vi "Process.vi"(8 "error in (no error)":errorcluster, 11 "SMO.UI.Example":refnum<class "SMO.UI.Example.lvclass">) -> (0 "error out":errorcluster, 3 "SMO.UI.Example out":refnum<class "SMO.UI.Example.lvclass">)   [LabVIEW 2013, in "SMO.UI.Example.lvclass"]
uses:
  SMO.UI.Example.lvclass
  SMO/Typedefs/Parent Call--Enum.ctl
  SMO.UI.Example.lvclass/SMO.UI.Example.ctl
  SMO.UI/SMO.UI.lvclass
  <vilib>/Utility/miscctls.llb/LVPointTypeDef.ctl
  SMO.Example/SMO.Example.lvclass
  SMO/SMO.lvclass
panel:
  in  "------------ User Events -------":bool=TRUE
  out "Waveform Chart":cluster{"Flow 2":dbl, "Flow 1":dbl}(graph)
  out "Sensor 1 (LPM)":u8
  out "Sensor 2 (LPM)":u8
  in  "Valve":bool
  in  "Pump":bool
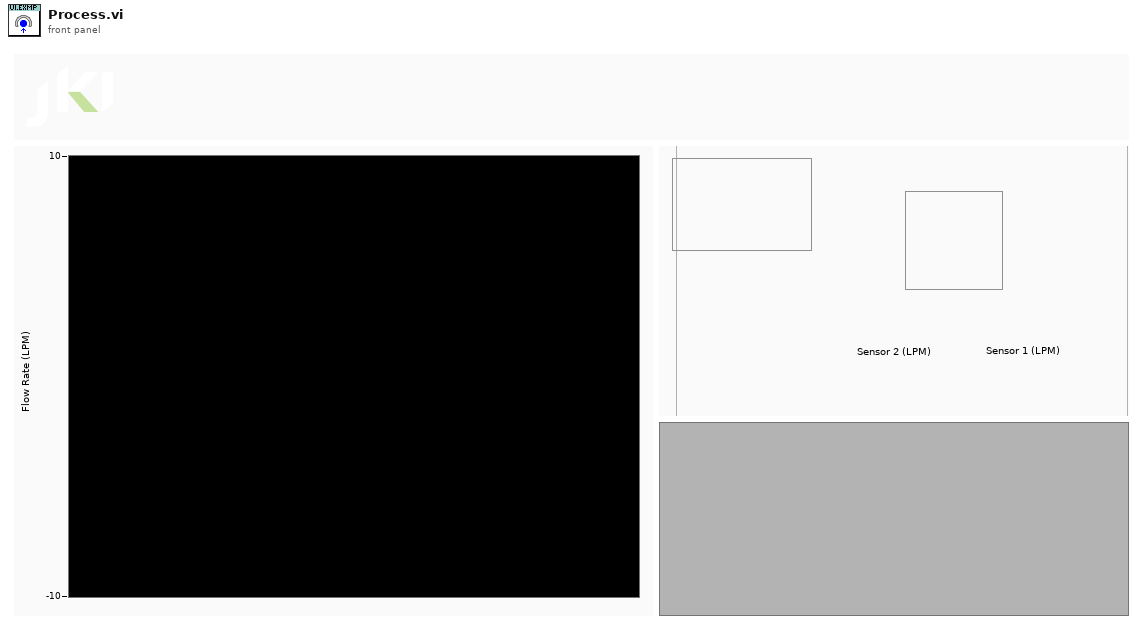
[diagram p1: front panel]
types:
  T1 = typedef "SMO.lvclass/Parent Call--Enum.ctl" = enum16{"Allows parent to run", "Does not request parent to run"}
  T2 = enum32{"invalid app kind", "Development System", "Run Time System", "Student Edition", "Embedded LabVIEW", "Evaluation", "Custom"}
  T3 = typedef "LVPointTypeDef.ctl" = cluster{"Horizontal":i16, "Vertical":i16}
  T4 = enum32{"Invalid", "Standard", "Closed", "Hidden", "Minimized", "Maximized"}
  T5 = typedef "SMO.UI.Example.lvclass/Dependencies--Cluster.ctl" = cluster{"SMO.Example":refnum<class "SMO.Example.lvclass">}
  T6 = cluster{"Core":cluster{"Current VI Reference":refnum<vi>, "Close Panel on Exit?":bool, "error":errorcluster}, "Self Ref":refnum<class "SMO.UI.Example.lvclass">, "Dependencies":T5, "Flow 1":dbl, "Flow 2":dbl}
  T7 = cluster{"Current VI Reference":refnum<vi>, "Close Panel on Exit?":bool, "error":errorcluster}
  T8 = typedef "SMO.lvclass/Protected Events.ctl" = cluster{"StopProcesses":refnum<user-event>, "AbortProcesses":refnum<user-event>}
  T9 = cluster{"Event Registration Refnum":refnum<event-registration>, "SMO.Example Public Events":refnum<event-registration>}
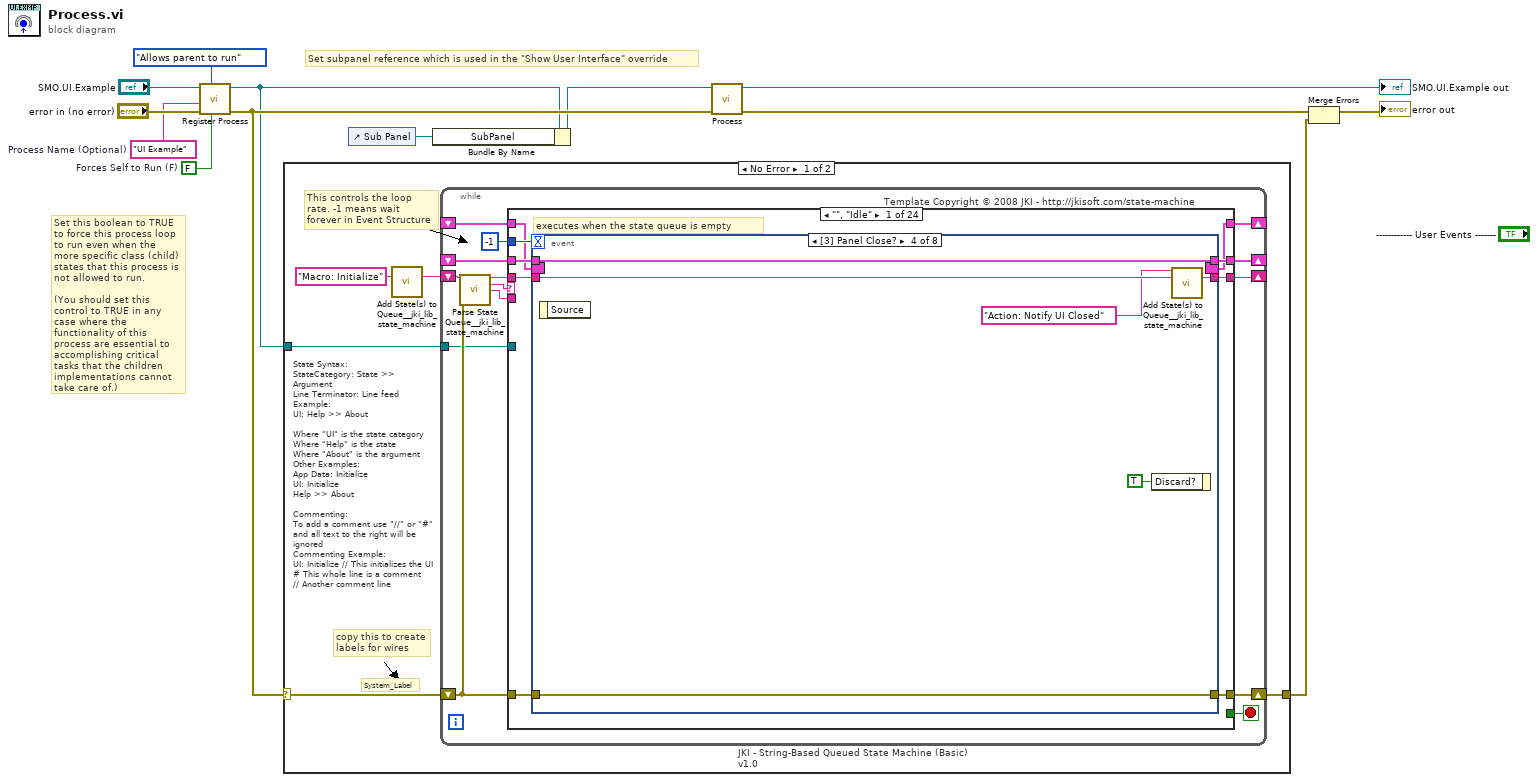
[diagram p0: block diagram]
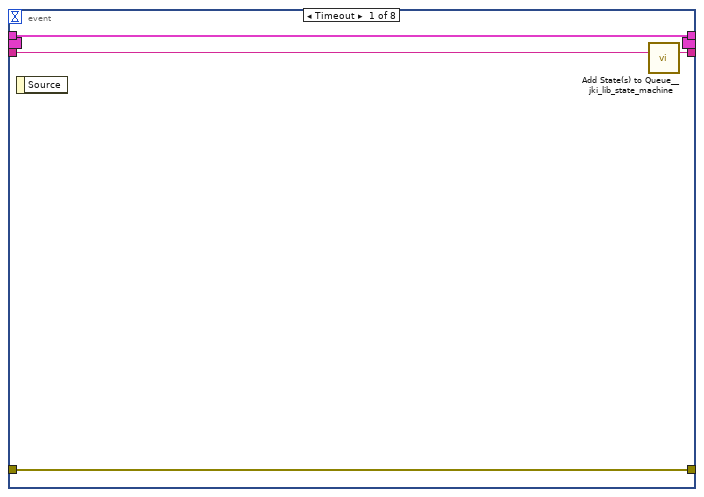
[diagram p2: hidden frame]
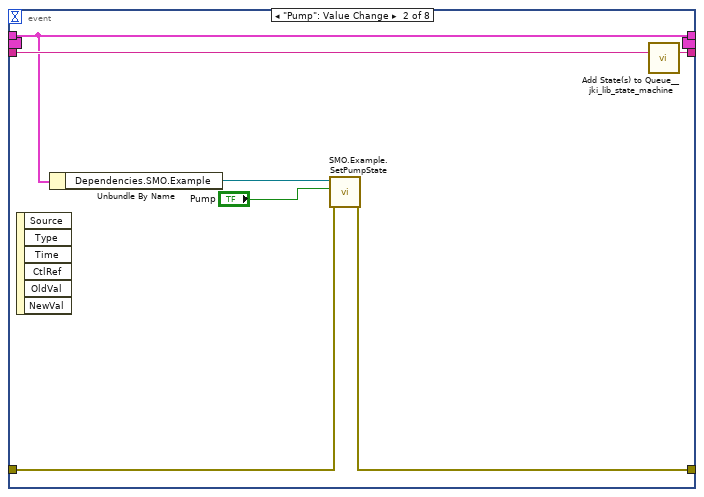
[diagram p3: hidden frame]
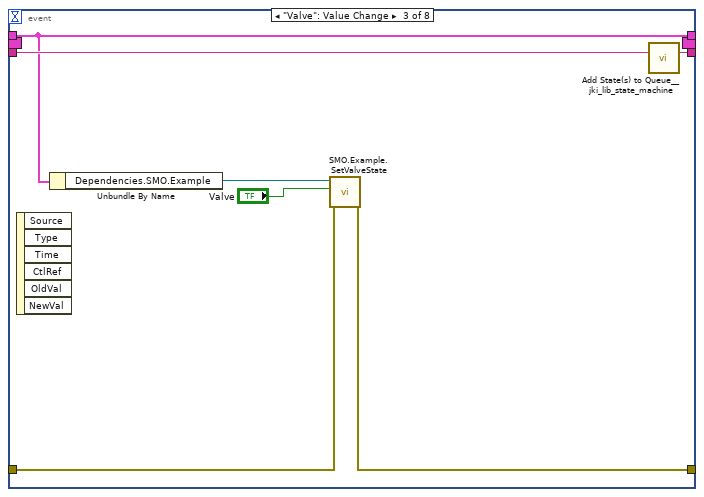
[diagram p4: hidden frame]
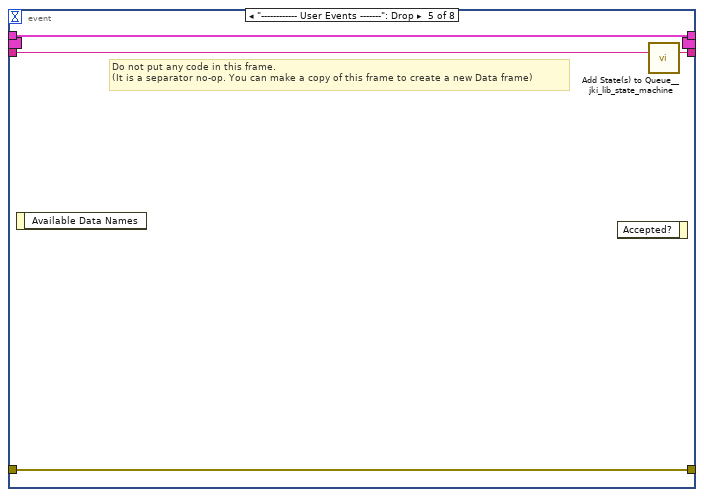
[diagram p5: hidden frame]
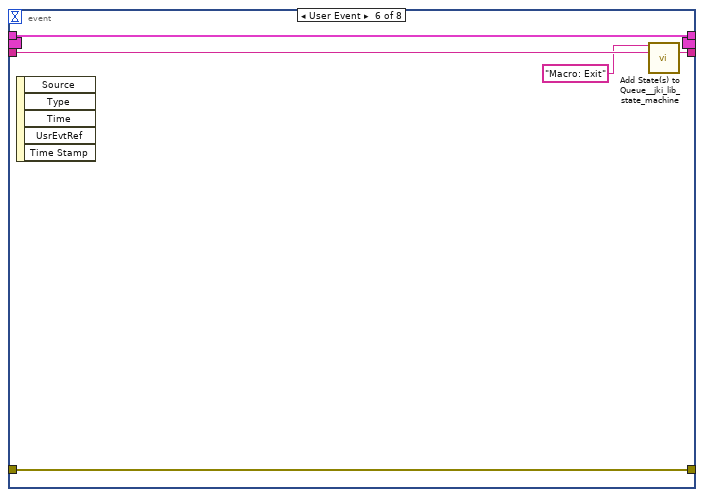
[diagram p6: hidden frame]
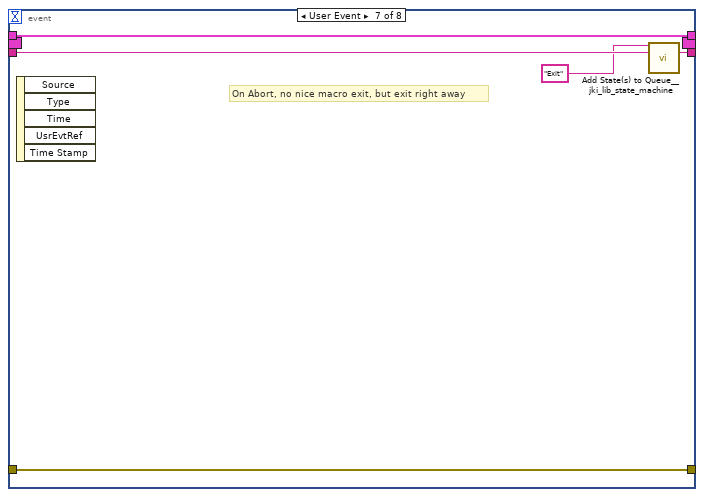
[diagram p7: hidden frame]
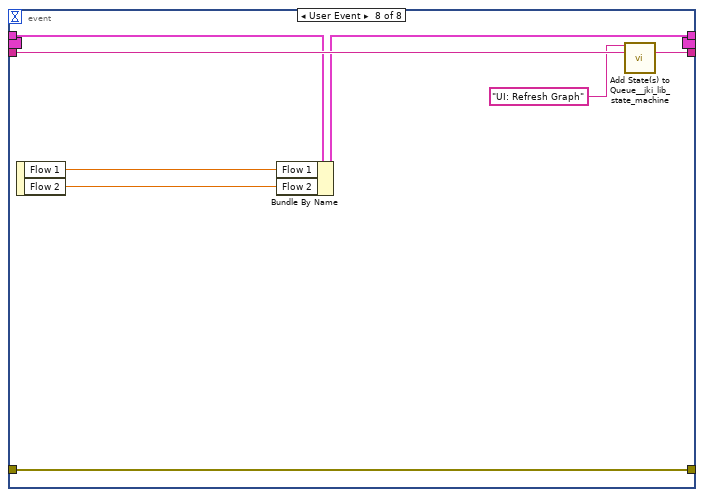
[diagram p8: hidden frame]
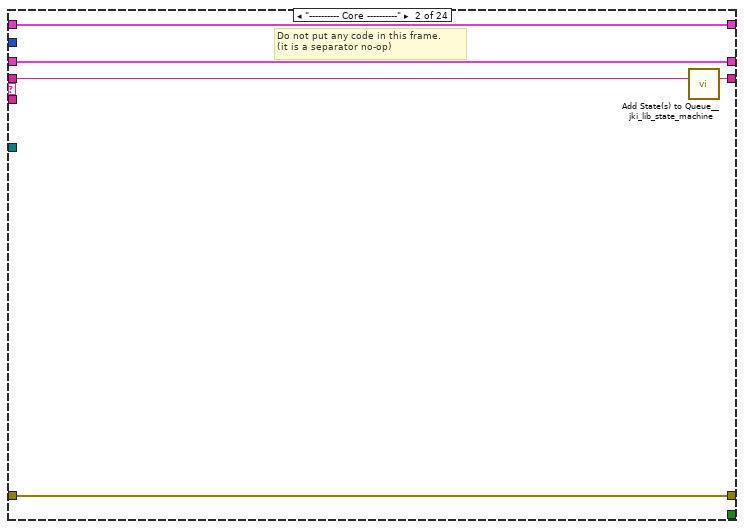
[diagram p9: hidden frame]
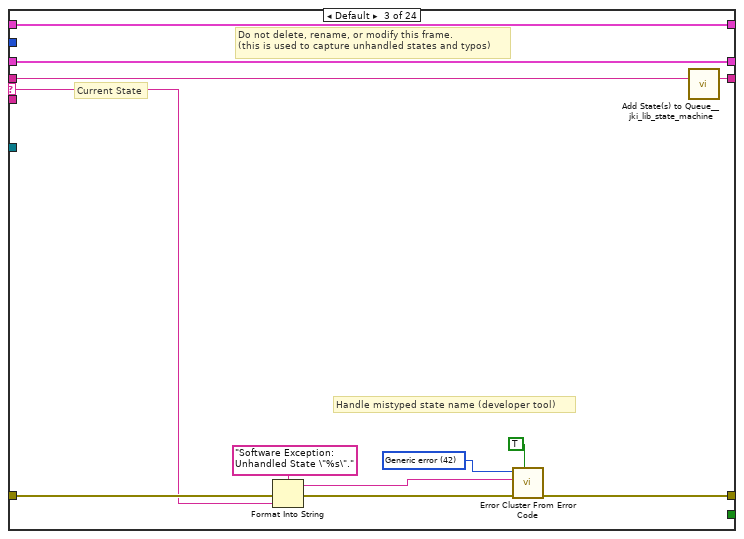
[diagram p10: hidden frame]
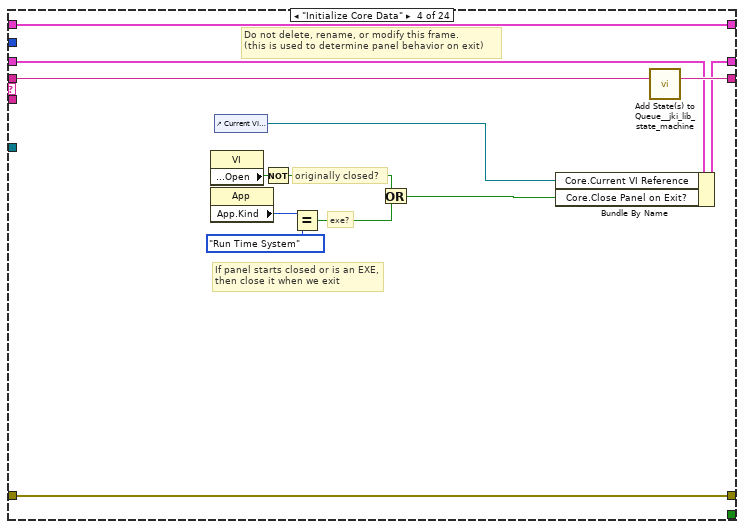
[diagram p11: hidden frame]
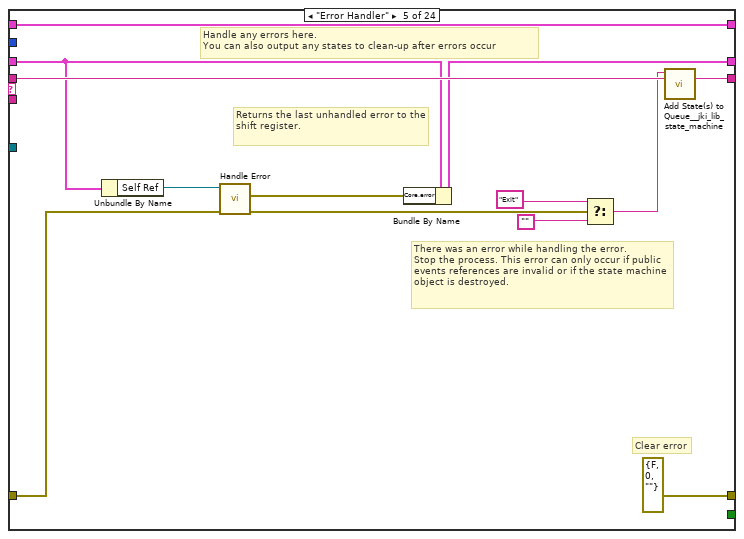
[diagram p12: hidden frame]
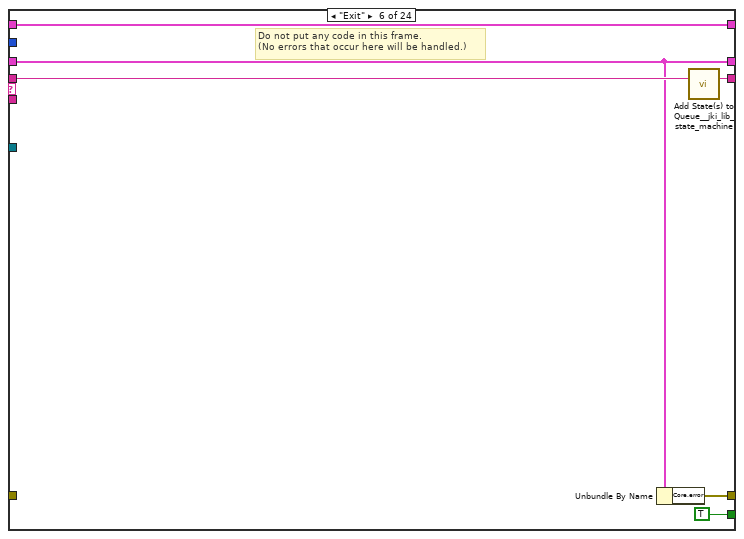
[diagram p13: hidden frame]
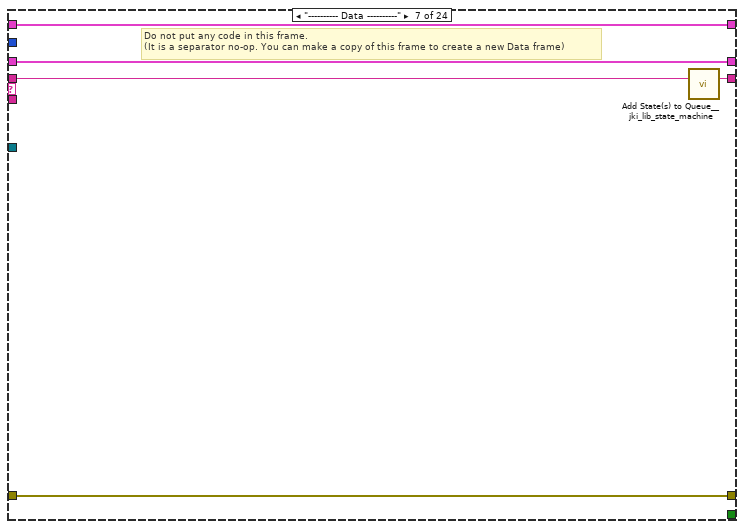
[diagram p14: hidden frame]
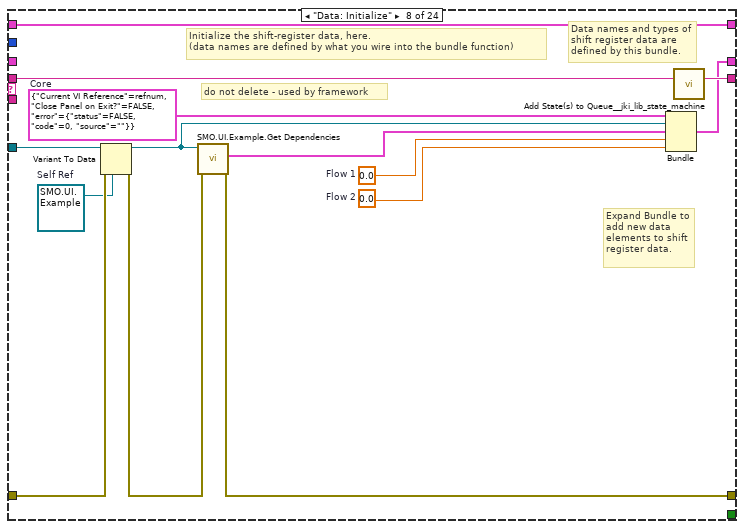
[diagram p15: hidden frame]
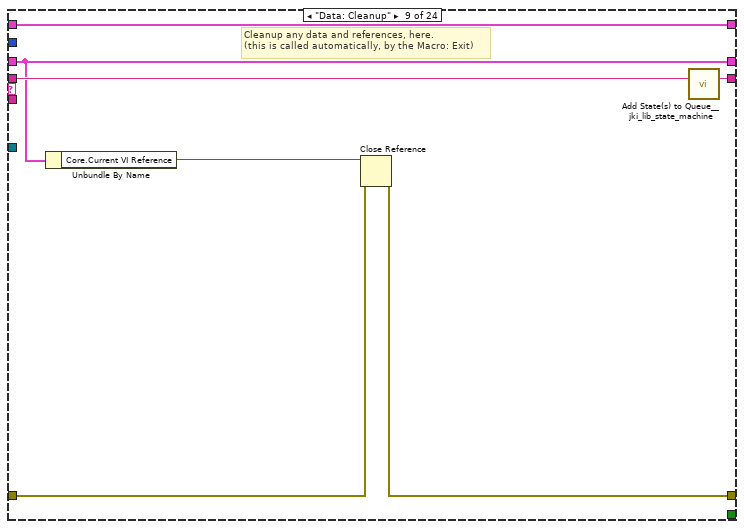
[diagram p16: hidden frame]
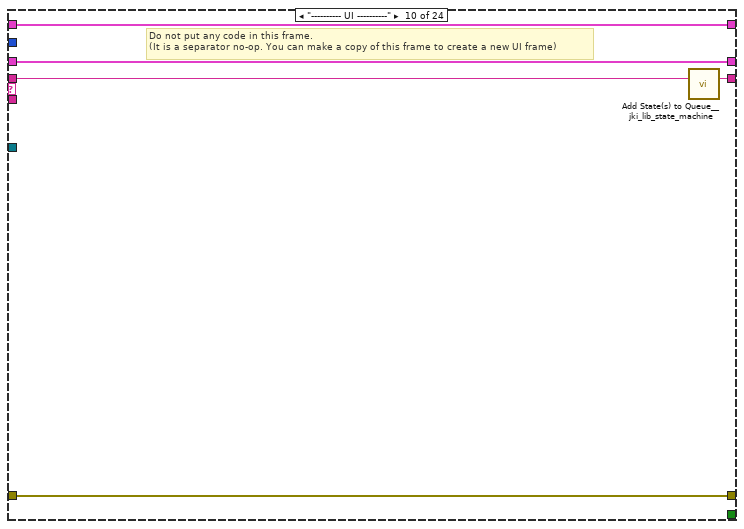
[diagram p17: hidden frame]
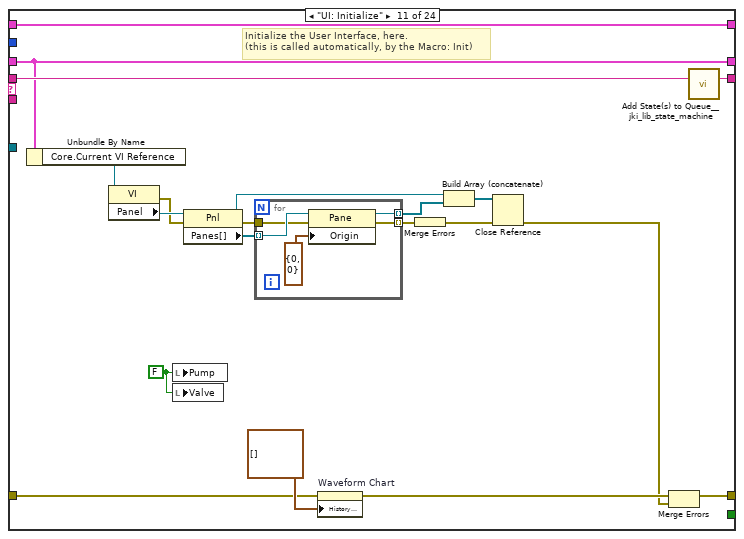
[diagram p18: hidden frame]
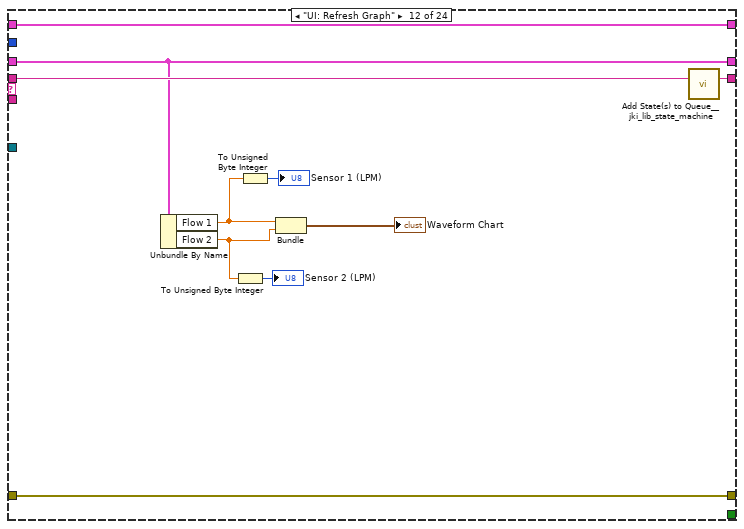
[diagram p19: hidden frame]
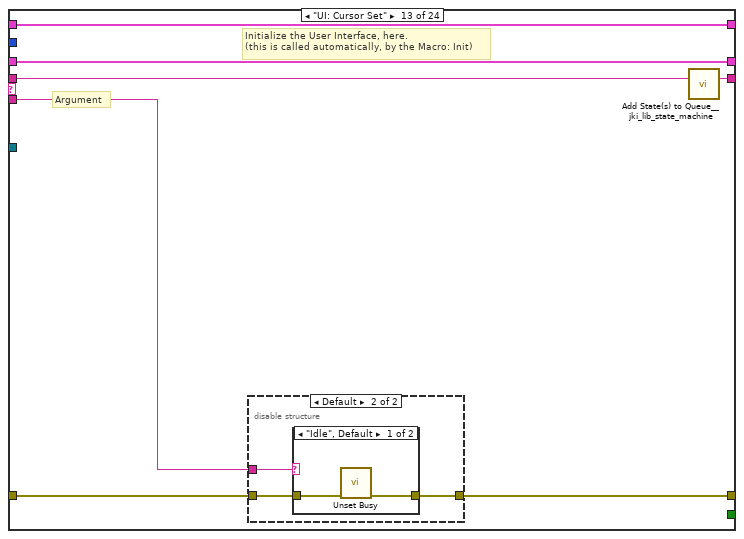
[diagram p20: hidden frame]
diagram:
  w1 = FALSE  # Forces Self to Run (F)
  w6 = "UI Example"  # Process Name (Optional)
  # "Set this boolean to TRUE to force this process loop to run even when the more specific class (child) states that this process is not allowed to run.\n\n(You should set this control to TRUE in any case where the functionality of this process are essential to accomplishing critical tasks that the children implementations cannot take care of.)"
  # "Set subpanel reference which is used in the \"Show User Interface\" override"
  n1 = call "Register Process.vi"("Forces Self to Run (F)"=w1, "Parent Call"=Parent_Call--Enum."Allows parent to run", "error in (no error)"="error in (no error)", "Process Name (optional)"=w6, "SMO"="SMO.UI.Example") -> ("error out"=w13:errorcluster, "SMO out"=w4:refnum<class "SMO.UI.Example.lvclass">)  [unwired: 5 in]
  n2 = case shown="No Error" w13 {
    selector: w13 -> [w15 w334]
    tunnel: w4 -> [w16 _]
    tunnel: [w14 w334] -> w11
    frame No Error {
      # "State Syntax:\nStateCategory: State >> Argument\nLine Terminator: Line feed\nExample:\nUI: Help >> About\n\nWhere \"UI\" is the state category\nWhere \"Help\" is the state\nWhere \"About\" is the argument\nOther Examples:\nApp Data: Initialize\nUI: Initialize\nHelp >> About\n\nCommenting:\nTo add a comment use \"//\" or \"#\" and all text to the right will be ignored\nCommenting Example:\nUI: Initialize // This initializes the UI\n# This whole line is a comment\n// Another comment line"
      # "copy this to create labels for wires"
      # "This controls the loop rate. -1 means wait forever in Event Structure"
      # "System_Label"
      n3 = call <vilib>:"Add State(s) to Queue__jki_lib_state_machine.vi"("State(s) in (\"\")"="Macro: Initialize") -> ("States Out"=w18:string)  [unwired: 14 in]
      n4 = while "JKI - String-Based Queued State Machine (Basic) v1.0" {
        shift-right: [w25] -> _
        shift-left: _ -> [w24]
        shift-right: [w28] -> w14
        shift-left: w15 -> [w22]
        shift-right: [w27] -> _
        shift-left: w18 -> [w29]
        tunnel: w16 -> [w21]
        shift-right: [w20] -> _
        shift-left: _ -> [w19]
        stop <- w26 stop-if-true
        # "Template Copyright © 2008 JKI - http://jkisoft.com/state-machine"
        n5 = call <vilib>:"Parse State Queue__jki_lib_state_machine.vi"("State Queue"=w29, "Error In (no error)"=w22) -> ("Remaining States"=w31:string, "Current State"=w32:string, "Arguments"=w30:string)  [unwired: 11 in]
        n6 = case shown="\"\", \"Idle\"" w32 {
          selector: w32 -> [_ _ w94 _ _ _ _ _ _ _ _ _ _ _ _ _ _ _ _ _ _ _ _ _]
          tunnel: w31 -> [w41 w92 w98 w117 w130 w136 w141 w155 w162 w167 w187 w202 w209 w225 w257 w266 w280 w285 w296 w301 w316 w321 w326 w333]
          tunnel: w30 -> [_ _ _ _ _ _ _ _ _ _ _ _ w203 w221 _ _ _ _ _ _ _ _ _ _]
          tunnel: w24 -> [w39 w89 w96 w108 w119 w132 w138 _ w157 w164 w182 w194 w207 w223 w254 w262 w271 w282 w293 w298 w314 w319 w323 w329]
          tunnel: [w38 w90 w100 w114 errorcluster {"status"=FALSE, "code"=0, "source"=""} ("error out") w131 w139 w144 w158 w165 w173 w193 w204 w218 w255 w264 w278 w283 w287 w299 w306 w318 w324 w327] -> w28
          tunnel: w22 -> [w37 w90 w99 w114 w121 _ w139 w152 w159 w165 w176 w193 w205 w219 w255 w264 w278 w283 w288 w299 w307 w318 w324 w328]
          tunnel: [w40 w91 w97 w116 w129 w135 w140 w154 w161 w166 w186 w201 w208 w224 w256 w265 w279 w284 w295 w300 w315 w320 w325 w332] -> w27
          tunnel: [_ _ _ _ _ TRUE _ _ _ _ _ _ _ _ _ _ _ _ _ _ _ _ _ _] -> w26
          tunnel: [w36 w89 w96 w115 w118 w132 w138 w153 w157 w164 w182 w194 w207 w223 w254 w262 w271 w282 w293 w298 w314 w319 w323 w329] -> w25
          tunnel: -1 ("Timeout") -> [w35 _ _ _ _ _ _ _ _ _ _ _ _ _ _ _ _ _ _ _ _ _ _ _]
          tunnel: w21 -> [_ _ _ _ _ _ _ w151 _ _ _ _ _ _ _ _ _ _ _ _ _ _ _ _]
          tunnel: [w33 w88 w93 w105 w127 w133 w137 w150 w156 w163 w183 w200 w206 w222 w253 w263 w272 w281 w294 w297 w309 w317 w322 w331] -> w20
          tunnel: w19 -> [w34 w88 w93 w105 w127 w133 w137 w150 w156 w163 w183 w200 w206 w222 w253 w263 w272 w281 w294 w297 _ w317 w322 w331]
          frame "", "Idle" {
            # "executes when the state queue is empty"
            n7 = event shown="[3] Panel Close?" {
              selector: w34 -> [_ _ _ _ _ _ _ _]
              dyn-events: [_ _ _ _ _ _ _ _] -> w33
              timeout: w35 -> [_ _ _ _ _ _ _ _]
              tunnel: w41 -> [w45 w52 w59 w65 w69 w74 w79 w87]
              tunnel: [w44 w51 w58 w64 w68 w73 w78 w86] -> w40
              tunnel: w39 -> [w42 w50 w57 w63 w66 w71 w76 w83]
              tunnel: [w43 w46 w54 w61 w67 w72 w77 w85] -> w38
              tunnel: w37 -> [w43 w47 w55 w61 w67 w72 w77 w85]
              tunnel: [w42 w50 w57 w63 w66 w71 w76 w84] -> w36
              event Timeout {
                n8 = event-data() -> ()  [unwired: 1 in, 1 out]
                n9 = call <vilib>:"Add State(s) to Queue__jki_lib_state_machine.vi"("State(s) in (\"\")"=w45) -> ("States Out"=w44:string)  [unwired: 14 in]
              }
              event "Pump": Value Change {
                n10 = event-data() -> ()  [unwired: 1 in, 6 out]
                n11 = Unbundle By Name(w50) -> ("Dependencies.SMO.Example"=w49:refnum<class "SMO.Example.lvclass">)
                n12 = call "SMO.Example.SetPumpState.vi"("error in (no error)"=w47, "Pump State"="Pump", "SMO.Example"=w49) -> ("error out"=w46:errorcluster)  [unwired: 7 in, 1 out]
                n13 = call <vilib>:"Add State(s) to Queue__jki_lib_state_machine.vi"("State(s) in (\"\")"=w52) -> ("States Out"=w51:string)  [unwired: 14 in]
              }
              event "Valve": Value Change {
                n14 = event-data() -> ()  [unwired: 1 in, 6 out]
                n15 = Unbundle By Name(w57) -> ("Dependencies.SMO.Example"=w56:refnum<class "SMO.Example.lvclass">)
                n16 = call "SMO.Example.SetValveState.vi"("error in (no error)"=w55, "Valve State"="Valve", "SMO.Example"=w56) -> ("error out"=w54:errorcluster)  [unwired: 7 in, 1 out]
                n17 = call <vilib>:"Add State(s) to Queue__jki_lib_state_machine.vi"("State(s) in (\"\")"=w59) -> ("States Out"=w58:string)  [unwired: 14 in]
              }
              event Panel Close? {
                n18 = event-data() -> ()  [unwired: 1 in, 1 out]
                n19 = event-data("Discard?"=TRUE) -> ()  [unwired: 1 in, 1 out]
                n20 = call <vilib>:"Add State(s) to Queue__jki_lib_state_machine.vi"("State(s) in Front (\"\")"="Action: Notify UI Closed" ("State(s) in Front (\"\")"), "State(s) in (\"\")"=w65) -> ("States Out"=w64:string)  [unwired: 13 in]
              }
              event "------------ User Events -------": Drop {
                # "Do not put any code in this frame.\n(It is a separator no-op. You can make a copy of this frame to create a new Data frame)"
                n21 = event-data() -> ()  [unwired: 1 in, 1 out]
                n22 = event-data() -> ()  [unwired: 2 in, 1 out]
                n23 = call <vilib>:"Add State(s) to Queue__jki_lib_state_machine.vi"("State(s) in (\"\")"=w69) -> ("States Out"=w68:string)  [unwired: 14 in]
              }
              event User Event {
                n24 = event-data() -> ()  [unwired: 1 in, 5 out]
                n25 = call <vilib>:"Add State(s) to Queue__jki_lib_state_machine.vi"("State(s) in Front (\"\")"="Macro: Exit", "State(s) in (\"\")"=w74) -> ("States Out"=w73:string)  [unwired: 13 in]
              }
              event User Event {
                # "On Abort, no nice macro exit, but exit right away"
                n26 = event-data() -> ()  [unwired: 1 in, 5 out]
                n27 = call <vilib>:"Add State(s) to Queue__jki_lib_state_machine.vi"("State(s) in Front (\"\")"="Exit", "State(s) in (\"\")"=w79) -> ("States Out"=w78:string)  [unwired: 13 in]
              }
              event User Event {
                n28 = event-data() -> ("Flow 1"=w82:dbl, "Flow 2"=w81:dbl)  [unwired: 1 in]
                n29 = Bundle By Name(cluster=w83, "Flow 1"=w82, "Flow 2"=w81) -> (w84:T6)
                n30 = call <vilib>:"Add State(s) to Queue__jki_lib_state_machine.vi"("State(s) in Front (\"\")"="UI: Refresh Graph", "State(s) in (\"\")"=w87) -> ("States Out"=w86:string)  [unwired: 13 in]
              }
            }
          }
          frame "---------- Core ----------" {
            # "Do not put any code in this frame.\n(it is a separator no-op)"
            n31 = call <vilib>:"Add State(s) to Queue__jki_lib_state_machine.vi"("State(s) in (\"\")"=w92) -> ("States Out"=w91:string)  [unwired: 14 in]
          }
          frame Default {
            w103 = 42 items=["No error", "Argument error", "Memory is full", "Out of zone", "End of file", "File already open", "Generic file I/O error", "File not found", "File permission error", "Disk is full", "Duplicate path", "Too many files open", "System feature not enabled", "Resource file not found", "Cannot add resource", "Resource not found", "Image not found", "Image memory error", "Pen does not exist", "Config type invalid", "Config token not found", "Config parse error", "Config memory error", "Bad external code format", "Bad external code offset", "External code not present", "Null window", "Destroy window error", "Null menu", "Print aborted", "Bad print record", "Print driver error", "Windows error during printing", "Memory error during printing", "Print dialog error", "Generic print error", "Invalid device refnum", "Device not found", "Device parameter error", "Device unit error", "Cannot open device", "Device call aborted", "Generic error", "Cancelled by user", "Object ID too low", "Object ID too high", "Object not in heap", "Unknown heap", "Unknown object (invalid DefProc)", "Unknown object (DefProc not in table)", "Message out of range", "Invalid (null) method", "Unknown message", "Manager call not supported", "Bad address", "Network operation in progress", "Network operation timed out", "Connection is busy", "Network attribute not supported", "Network error", "Address in use", "System out of memory", "Connection aborted", "Connection refused", "Not connected", "Already connected", "Connection closed", "Initialization error (interapplication manager)", "Bad occurrence", "Wait on unbound occurrence handler", "Occurrence queue overflow", "Datalog type conflict", "Unused", "Unrecognized type (interapplication manager)", "Memory corrupt", "Failed to make temporary DLL", "Old CIN version", "Drag socket not found", "Failed to load drop-object", "Failed to register OLE object", "Failed to release OLE object", "Format specifier type mismatch", "Unknown format specifier", "Too few format specifiers", "Too many format specifiers", "Scan failed", "Newer CIN version", "Error converting to variant", "Runtime menu error", "Password tampered", "Variant attribute not found", "Incompatible variant data type", "Event data is not available", "Event Store is not present", "Occurrence is not found", "Event Queue is not created", "Event info is not available", "Refnum passed is NULL", "Error retrieving Class GUID", "Error retrieving CoClass GUID", "Error retrieving TypeLib GUID.", "Bad built application magic bytes.", "Specific driver is different from the specific driver associated with the Logical Name.", "There is no session opened to the class driver.", "Max Error", "MAX - Error with config objects", "MAX - Error loading configuration", "MAX - Group not supported"]
            # "Current State"
            # "Do not delete, rename, or modify this frame.\n(this is used to capture unhandled states and typos)"
            # "Handle mistyped state name (developer tool)"
            n32 = Format Into String(format string="Software Exception: Unhandled State \"%s\"." ("message"), error in=w99, w94) -> (resulting string=w102:string, error out=w101:errorcluster)  [unwired: 1 in]
            n33 = call <vilib>:"Error Cluster From Error Code.vi"("show call chain? (False)"=TRUE, "error in (no error)"=w101, "error message (\"\")"=w102, "error code (0)"=w103) -> ("error out"=w100:errorcluster)  [unwired: 5 in]
            n34 = call <vilib>:"Add State(s) to Queue__jki_lib_state_machine.vi"("State(s) in (\"\")"=w98) -> ("States Out"=w97:string)  [unwired: 14 in]
          }
          frame "Initialize Core Data" {
            # "Do not delete, rename, or modify this frame.\n(this is used to determine panel behavior on exit)"
            # "originally closed?"
            # "exe?"
            # "If panel starts closed or is an EXE, then close it when we exit"
            n35 = property class="VI"() -> ("Front Panel.Open"=w113:bool)  [unwired: 2 in, 2 out]
            n36 = property class="App"() -> ("App.Kind"=w112:T2)  [unwired: 2 in, 2 out]
            n37 = control-ref of="Current VI Reference"() -> (w106:refnum<vi>)
            n38 = Not(x=w113) -> (.not. x?=w110:bool)
            n39 = Equal?(x=w112, y=T2."Run Time System" ("Application:Kind")) -> (x = y?=w109:bool)
            n40 = Or(x=w110, y=w109) -> (x .or. y?=w107:bool)
            n41 = Bundle By Name(cluster=w108, "Core.Current VI Reference"=w106, "Core.Close Panel on Exit?"=w107) -> (w115:T6)
            n42 = call <vilib>:"Add State(s) to Queue__jki_lib_state_machine.vi"("State(s) in (\"\")"=w117) -> ("States Out"=w116:string)  [unwired: 14 in]
          }
          frame "Error Handler" {
            # "Returns the last unhandled error to the shift register."
            # "There was an error while handling the error.\nStop the process. This error can only occur if public events references are invalid or if the state machine object is destroyed."
            # "Handle any errors here.\nYou can also output any states to clean-up after errors occur"
            # "Clear error"
            n43 = Unbundle By Name(w119) -> ("Self Ref"=w126:refnum<class "SMO.UI.Example.lvclass">)
            n44 = call-dynamic "Handle Error.vi"("error in"=w121, "SMO"=w126) -> ("handling error"=w124:errorcluster, "Unhandled error"=w125:errorcluster)  [unwired: 7 in, 1 out]
            n45 = Bundle By Name(cluster=w119, "Core.error"=w125) -> (w118:T6)
            n46 = Select(t="Exit", s=w124, f="") -> (s? t:f=w120:string)
            n47 = call <vilib>:"Add State(s) to Queue__jki_lib_state_machine.vi"("State(s) in Front (\"\")"=w120, "State(s) in (\"\")"=w130) -> ("States Out"=w129:string)  [unwired: 13 in]
          }
          frame "Exit" {
            # "Do not put any code in this frame.\n(No errors that occur here will be handled.)"
            n48 = Unbundle By Name(w132) -> ("Core.error"=w131:errorcluster)
            n49 = call <vilib>:"Add State(s) to Queue__jki_lib_state_machine.vi"("State(s) in (\"\")"=w136) -> ("States Out"=w135:string)  [unwired: 14 in]
          }
          frame "---------- Data ----------" {
            # "Do not put any code in this frame.\n(It is a separator no-op. You can make a copy of this frame to create a new Data frame)"
            n50 = call <vilib>:"Add State(s) to Queue__jki_lib_state_machine.vi"("State(s) in (\"\")"=w141) -> ("States Out"=w140:string)  [unwired: 14 in]
          }
          frame "Data: Initialize" {
            w143 = 0.0  # Flow 1
            w142 = 0.0  # Flow 2
            w148 = refnum<class "SMO.UI.Example.lvclass"> refnum  # Self Ref
            w149 = T7 {"Current VI Reference"=refnum, "Close Panel on Exit?"=FALSE, "error"={"status"=FALSE, "code"=0, "source"=""}}  # Core
            # "do not delete - used by framework"
            # "Expand Bundle to add new data elements to shift register data."
            # "Data names and types of shift register data are defined by this bundle."
            # "Initialize the shift-register data, here.\n(data names are defined by what you wire into the bundle function)"
            n51 = Variant To Data(error in=w152, type=w148, Variant=w151) -> (data=w146:refnum<class "SMO.UI.Example.lvclass">, error out=w145:errorcluster)
            n52 = call "SMO.UI.Example.Get Dependencies.vi"("error in (no error)"=w145, "SMO UI.Template in"=w146) -> ("error out"=w144:errorcluster, "Dependencies"=w147:T5)  [unwired: 7 in, 1 out]
            n53 = Bundle("Core"=w149, "Self Ref"=w146, "Dependencies"=w147, "Flow 1"=w143, "Flow 2"=w142) -> (w153:T6)  [unwired: 1 in]
            n54 = call <vilib>:"Add State(s) to Queue__jki_lib_state_machine.vi"("State(s) in (\"\")"=w155) -> ("States Out"=w154:string)  [unwired: 14 in]
          }
          frame "Data: Cleanup" {
            # "Cleanup any data and references, here.\n(this is called automatically, by the Macro: Exit)"
            n55 = Unbundle By Name(w157) -> ("Core.Current VI Reference"=w160:refnum<vi>)
            n56 = Close Reference(reference=w160, error in (no error)=w159) -> (error out=w158:errorcluster)
            n57 = call <vilib>:"Add State(s) to Queue__jki_lib_state_machine.vi"("State(s) in (\"\")"=w162) -> ("States Out"=w161:string)  [unwired: 14 in]
          }
          frame "---------- UI ----------" {
            # "Do not put any code in this frame.\n(It is a separator no-op. You can make a copy of this frame to create a new UI frame)"
            n58 = call <vilib>:"Add State(s) to Queue__jki_lib_state_machine.vi"("State(s) in (\"\")"=w167) -> ("States Out"=w166:string)  [unwired: 14 in]
          }
          frame "UI: Initialize" {
            w185 = FALSE ("Pump")
            # "Initialize the User Interface, here.\n(this is called automatically, by the Macro: Init)"
            n59 = Unbundle By Name(w182) -> ("Core.Current VI Reference"=w181:refnum<vi>)
            n60 = property class="VI"(reference=w181) -> (error out=w178:errorcluster, "Panel"=w180:refnum<vi>)  [unwired: 1 in, 1 out]
            n61 = local write "Pump"(w185) -> ()
            n62 = local write "Valve"(w185) -> ()
            n63 = property class="Pnl"(reference=w180, error in=w178) -> (reference out=w172:refnum<vi>, error out=w177:errorcluster, "Panes[]"=w179:refnum<vi>[])
            n64 = for {
              tunnel: w179 -> [w192] mode=indexing
              tunnel: w177 -> [w190]
              tunnel: [w189] -> w175 mode=indexing
              tunnel: [w188] -> w171 mode=indexing
              n65 = property class="Pane"(reference=w192, error in=w190, "Origin"=T3 {"Horizontal"=0, "Vertical"=0}) -> (reference out=w188:refnum<vi>, error out=w189:errorcluster)
            }
            n66 = property on="Waveform Chart" class="WFChart (strict)"(error in=w176, "History Data"=cluster{"Flow 2":dbl, "Flow 1":dbl}[] []) -> (error out=w174:errorcluster)  [unwired: 1 in, 1 out]
            n67 = Merge Errors(w175) -> (w170:errorcluster)
            n68 = Build Array (concatenate)(w172, w171) -> (w168:refnum<vi>[])
            n69 = Close Reference(reference=w168, error in (no error)=w170) -> (error out=w169:errorcluster)
            n70 = Merge Errors(w174, w169) -> (w173:errorcluster)
            n71 = call <vilib>:"Add State(s) to Queue__jki_lib_state_machine.vi"("State(s) in (\"\")"=w187) -> ("States Out"=w186:string)  [unwired: 14 in]
          }
          frame "UI: Refresh Graph" {
            n72 = Unbundle By Name(w194) -> ("Flow 1"=w197:dbl, "Flow 2"=w198:dbl)
            n73 = To Unsigned Byte Integer(number=w198) -> (unsigned 8bit integer=→"Sensor 2 (LPM)":u8)
            n74 = To Unsigned Byte Integer(number=w197) -> (unsigned 8bit integer=→"Sensor 1 (LPM)":u8)
            n75 = Bundle("Flow 1"=w197, "Flow 2"=w198) -> (→"Waveform Chart":cluster{"Flow 1":dbl, "Flow 2":dbl})  [unwired: 1 in]
            n76 = call <vilib>:"Add State(s) to Queue__jki_lib_state_machine.vi"("State(s) in (\"\")"=w202) -> ("States Out"=w201:string)  [unwired: 14 in]
          }
          frame "UI: Cursor Set" {
            # "Argument"
            # "Initialize the User Interface, here.\n(this is called automatically, by the Macro: Init)"
            n77 = disable-structure shown="Default" {
              disable-tunnel: w205 -> [w210 w213]
              disable-tunnel: [w210 w212] -> w204
              disable-tunnel: w203 -> [_ w211]
              frame condition #0 {
              }
              frame condition #1 (active) {
                n78 = case shown="\"Idle\", Default" w211 {
                  tunnel: w213 -> [w215 w217]
                  tunnel: [w214 w216] -> w212
                  frame "Idle", Default {
                    n79 = call <vilib>:"Unset Busy.vi"("error in (no error)"=w215) -> ("error out"=w214:errorcluster)  [unwired: 10 in]
                  }
                  frame "Busy" {
                    n80 = call <vilib>:"Set Busy.vi"("error in (no error)"=w217) -> ("error out"=w216:errorcluster)  [unwired: 9 in, 1 out]
                  }
                }
              }
            }
            n81 = call <vilib>:"Add State(s) to Queue__jki_lib_state_machine.vi"("State(s) in (\"\")"=w209) -> ("States Out"=w208:string)  [unwired: 14 in]
          }
          frame "UI: Front Panel State" {
            # "Argument"
            # "Set Front Panel Open or Closed\n(Usage: \"UI: Front Panel State >> Open|Close\")"
            n82 = Unbundle By Name(w223) -> ("Core.Current VI Reference"=w220:refnum<vi>)
            n83 = disable-structure shown="Default" {
              disable-tunnel: w219 -> [w229 w252]
              disable-tunnel: [w228 w252] -> w218
              disable-tunnel: w220 -> [w227 _]
              disable-tunnel: w221 -> [w226 _]
              frame condition #0 (active) {
                n84 = case shown="\"Open\", Default" w226 {
                  tunnel: w229 -> [w233 w246]
                  tunnel: [w235 w247] -> w228
                  tunnel: w227 -> [w234 w244]
                  frame "Open", Default {
                    # "Open FP if not open or invalid"
                    n85 = property class="VI"(reference=w234, error in=w233) -> (reference out=w231:refnum<vi>, error out=w232:errorcluster, "FP.State"=w230:T4)
                    n86 = case shown="Default" w230 {
                      tunnel: [w238 w241] -> w235
                      tunnel: w232 -> [w237 w241]
                      tunnel: w231 -> [w236 _]
                      frame Default {
                        n87 = invoke class="VI" method="FP.Open"(reference=w236, error in=w237, "Activate"=TRUE, "State"=T4."Standard") -> (error out=w238:errorcluster)  [unwired: 1 in, 4 out]
                      }
                      frame "Invalid", "Standard" {
                      }
                    }
                  }
                  frame "Close" {
                    # "Close FP is not Closed or Invalid"
                    n88 = property class="VI"(reference=w244, error in=w246) -> (reference out=w243:refnum<vi>, error out=w245:errorcluster, "FP.State"=w242:T4)
                    n89 = case shown="Default" w242 {
                      tunnel: [w248 w251] -> w247
                      tunnel: w245 -> [w248 w250]
                      tunnel: w243 -> [_ w249]
                      frame "Invalid", "Closed" {
                      }
                      frame Default {
                        n90 = invoke class="VI" method="FP.Close"(reference=w249, error in=w250) -> (error out=w251:errorcluster)  [unwired: 1 in, 2 out]
                      }
                    }
                  }
                }
              }
              frame condition #1 {
              }
            }
            n91 = call <vilib>:"Add State(s) to Queue__jki_lib_state_machine.vi"("State(s) in (\"\")"=w225) -> ("States Out"=w224:string)  [unwired: 14 in]
          }
          frame "---------- Macro ----------" {
            # "Do not put any code in this frame.\n(It is a separator no-op. You can make a copy of this frame to create a new Macro frame)"
            n92 = call <vilib>:"Add State(s) to Queue__jki_lib_state_machine.vi"("State(s) in (\"\")"=w257) -> ("States Out"=w256:string)  [unwired: 14 in]
          }
          frame "Macro: Initialize" {
            w260 = "UI: Initialize\n//UI: Front Panel State >> Open"  # UI: Initialize //UI: Front Panel State >> Open
            # "Initialization Macro\n(This is called once, when the VI starts)"
            n93 = call <vilib>:"Add State(s) to Queue__jki_lib_state_machine.vi"("State(s) in Front (\"\")"="Data: Initialize\nInitialize Core Data\nEvents: Register", "State(s) in (\"\")"="Process: Sync", "State(s) at Back (\"\")"=w260) -> ("States Out"=w259:string)  [unwired: 12 in]
            n94 = call <vilib>:"Add State(s) to Queue__jki_lib_state_machine.vi"("State(s) in Front (\"\")"=w259, "State(s) in (\"\")"=w266) -> ("States Out"=w265:string)  [unwired: 13 in]
          }
          frame "Macro: Exit" {
            # "Exit Macro\n(This is called once, when the VI exits)"
            n95 = Unbundle By Name(w271) -> ("Core.Close Panel on Exit?"=w277:bool)
            n96 = Select(t="//UI: Front Panel State >> Close", s=w277, f="") -> (s? t:f=w274:string)
            n97 = call <vilib>:"Add State(s) to Queue__jki_lib_state_machine.vi"("State(s) in Front (\"\")"="Data: Cleanup\nEvents: Unregister", "State(s) in (\"\")"="Process: Sync", "State(s) at Back (\"\")"="Exit") -> ("States Out"=w268:string)  [unwired: 12 in]
            n98 = call <vilib>:"Add State(s) to Queue__jki_lib_state_machine.vi"("State(s) in (\"\")"=w274, "State(s) at Back (\"\")"=w268) -> ("States Out"=w273:string)  [unwired: 13 in]
            n99 = call <vilib>:"Add State(s) to Queue__jki_lib_state_machine.vi"("State(s) in Front (\"\")"=w273, "State(s) in (\"\")"=w280) -> ("States Out"=w279:string)  [unwired: 13 in]
          }
          frame "---------- Process ----------" {
            # "Template Separator\n(You can make a copy of, or modify, this frame)"
            n100 = call <vilib>:"Add State(s) to Queue__jki_lib_state_machine.vi"("State(s) in (\"\")"=w285) -> ("States Out"=w284:string)  [unwired: 14 in]
          }
          frame "Process: Sync" {
            n101 = Unbundle By Name(w293) -> ("Self Ref"=w289:refnum<class "SMO.UI.Example.lvclass">)
            n102 = call "WaitOnProcessSync.vi"("error in (no error)"=w288, "SMO"=w289) -> ("error out"=w287:errorcluster, "Don't run?"=w292:bool)  [unwired: 7 in, 1 out]
            n103 = Select(t="Data: Cleanup\nEvents: Unregister\nExit", s=w292, f="") -> (s? t:f=w286:string)
            n104 = call <vilib>:"Add State(s) to Queue__jki_lib_state_machine.vi"("State(s) in Front (\"\")"=w286, "State(s) in (\"\")"=w296) -> ("States Out"=w295:string)  [unwired: 13 in]
          }
          frame "---------- Events ----------" {
            # "Template Separator\n(You can make a copy of, or modify, this frame)"
            n105 = call <vilib>:"Add State(s) to Queue__jki_lib_state_machine.vi"("State(s) in (\"\")"=w301) -> ("States Out"=w300:string)  [unwired: 14 in]
          }
          frame "Events: Register" {
            # "Clear error when dependency not created. (Demo only)"
            # "Dependency Public Events"
            # "Base Class Protected Events"
            n106 = Unbundle By Name(w314) -> ("Self Ref"=w308:refnum<class "SMO.UI.Example.lvclass">)
            n107 = Unbundle By Name(w314) -> ("Dependencies.SMO.Example"=w312:refnum<class "SMO.Example.lvclass">)
            n108 = call "SMO.Example.GetPublicEventsRegistration.vi"("SMO.Example"=w312) -> ("error out"=w303:errorcluster, "SMO.Example Public Events"=w311:refnum<event-registration>)  [unwired: 8 in, 1 out]
            n109 = call <vilib>:"Clear Errors.vi"("error in (no error)"=w303) -> ("error out"=w302:errorcluster)  [unwired: 6 in]
            n110 = call "GetProtectedEvents.vi"("SMO"=w308) -> ("error out"=w304:errorcluster, "SMO Protected Events"=w313:T8)  [unwired: 8 in, 1 out]
            n111 = register-events(w313) -> (reference out=w310:refnum<event-registration>, error out=w305:errorcluster)  [unwired: 2 in]
            n112 = Merge Errors(w305, w304, w302, w307) -> (w306:errorcluster)
            n113 = Bundle("Event Registration Refnum"=w310, "SMO.Example Public Events"=w311) -> (w309:T9)  [unwired: 1 in]
            n114 = call <vilib>:"Add State(s) to Queue__jki_lib_state_machine.vi"("State(s) in (\"\")"=w316) -> ("States Out"=w315:string)  [unwired: 14 in]
          }
          frame "Events: Unregister" {
            # "Your code here.\n(You can make a copy of, or modify, this frame)"
            n115 = call <vilib>:"Add State(s) to Queue__jki_lib_state_machine.vi"("State(s) in (\"\")"=w321) -> ("States Out"=w320:string)  [unwired: 14 in]
          }
          frame "---------Action---------" {
            # "Action Separator\n(You can make a copy of, or modify, this frame)"
            n116 = call <vilib>:"Add State(s) to Queue__jki_lib_state_machine.vi"("State(s) in (\"\")"=w326) -> ("States Out"=w325:string)  [unwired: 14 in]
          }
          frame "Action: Notify UI Closed" {
            # "Notify that the UI has closed"
            # "Action Separator\n(You can make a copy of, or modify, this frame)"
            n117 = Unbundle By Name(w329) -> ("Self Ref"=w330:refnum<class "SMO.UI.Example.lvclass">)
            n118 = call "Hide.vi"("error in (no error)"=w328, "SMO.UI"=w330) -> ("error out"=w327:errorcluster)  [unwired: 8 in, 1 out]
            n119 = call <vilib>:"Add State(s) to Queue__jki_lib_state_machine.vi"("State(s) in (\"\")"=w333) -> ("States Out"=w332:string)  [unwired: 14 in]
          }
        }
      }
    }
    frame Error {
    }
  }
  n120 = control-ref of="Sub Panel"() -> (w2:refnum<vi>)
  n121 = Bundle By Name(cluster=w4, "SubPanel"=w2) -> (w3:refnum<class "SMO.UI.Example.lvclass">)
  n122 = call-parent "Process.vi"("error in (no error)"=w13, "SMO.UI"=w3) -> ("error out"=w12:errorcluster, "SMO.UI out"=→"SMO.UI.Example out":refnum<class "SMO.UI.Example.lvclass">)  [unwired: 8 in]
  n123 = Merge Errors(w12, w11) -> (→"error out":errorcluster)
